vi "Dynamic Dispatch Tester.vi"() -> ()   [LabVIEW 2010]
uses:
  Aggregate Sound/Aggregate Sound.lvclass
  Sound/Sound.lvclass
  <vilib>/Waveform/WDTOps.llb/WDT Append Waveforms DBL.vi
  Single Tone/Single Tone.lvclass
  Silence/Silence.lvclass
  Recorded Sound/Recorded Sound.lvclass
  Fade/Fade.lvclass
panel:
  out "Appended Waveforms":waveform(dbl)(graph)
  in  "Fade in? (True)":bool=TRUE
  in  "Silence Duration (1 second)":dbl=1.0
  in  "Tone Duration (1 second)":dbl=1.0
  in  "Frequency (500 Hz)":dbl=500.0
  # "Single Tone"
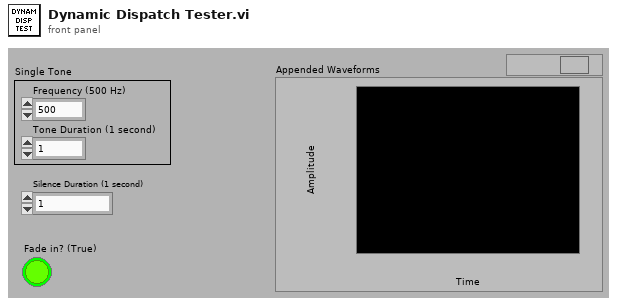
[diagram p1: front panel]
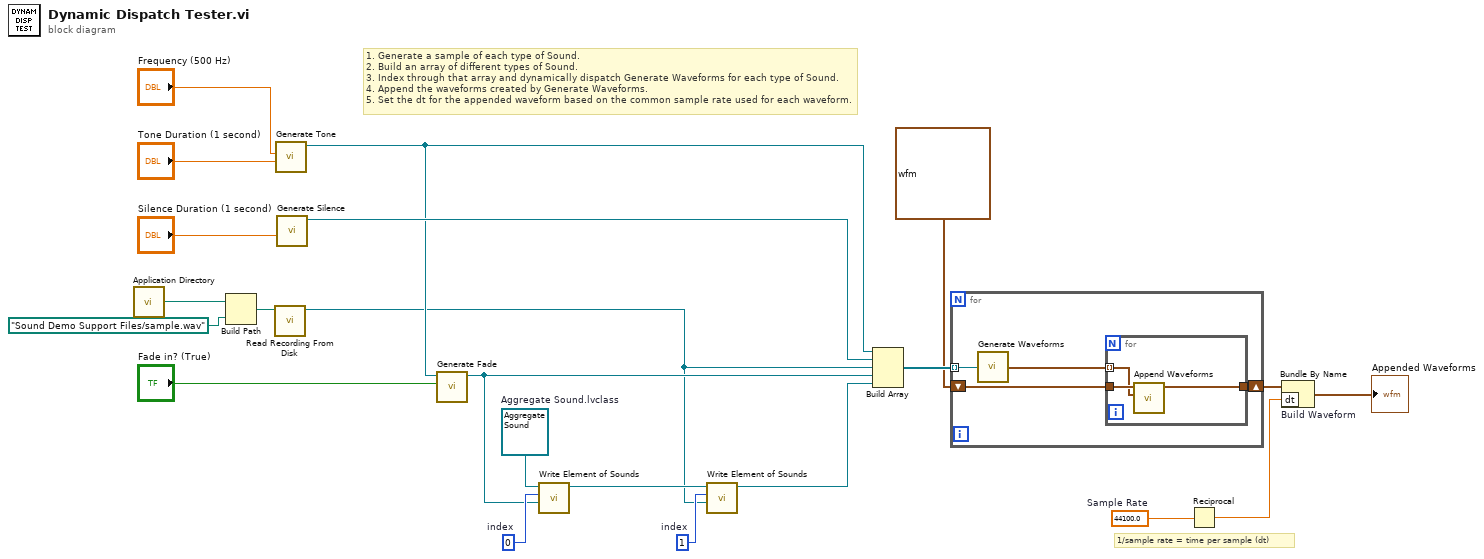
[diagram p0: block diagram]
diagram:
  w10 = 44100.0  # Sample Rate
  w15 = 1  # index
  w16 = 0  # index
  w18 = refnum<class "Aggregate Sound.lvclass"> refnum  # Aggregate Sound.lvclass
  # "1. Generate a sample of each type of Sound. \n2. Build an array of different types of Sound.\n3. Index through that array and dynamically dispatch Generate Waveforms for each type of Sound. \n4. Append the waveforms created by Generate Waveforms.\n5. Set the dt for the appended waveform based on the common sample rate used for each waveform."
  # "1/sample rate = time per sample (dt)"
  n1 = call <vilib>:"Application Directory.vi"() -> ("Application Directory"=w3:path)
  n2 = Build Path(base path=w3, name or relative path=path "Sound Demo Support Files/sample.wav" ("Recorded Sound Path")) -> (appended path=w1:path)
  n3 = call "Read Recording From Disk.vi"("File Path"=w1) -> ("Recorded Sound"=w4:refnum<class "Recorded Sound.lvclass">)  [unwired: 9 in, 1 out]
  n4 = call "Generate Tone.vi"("Duration (1 second)"="Tone Duration (1 second)", "Frequency (500 Hz)"="Frequency (500 Hz)") -> ("Single Tone out"=w5:refnum<class "Single Tone.lvclass">)  [unwired: 9 in]
  n5 = call "Generate Silence.vi"("Duration (1 second)"="Silence Duration (1 second)") -> ("Silence out"=w13:refnum<class "Silence.lvclass">)  [unwired: 10 in]
  n6 = call "Generate Fade.vi"("Fade in? (True)"="Fade in? (True)", "Original Sound"=w5) -> ("Fade"=w7:refnum<class "Fade.lvclass">)  [unwired: 9 in]
  n7 = call "Write Element of Sounds.vi"("Sound.lvclass"=w7, "index"=w16, "Aggregate Sound in"=w18) -> ("Aggregate Sound out"=w17:refnum<class "Aggregate Sound.lvclass">)  [unwired: 8 in]
  n8 = call "Write Element of Sounds.vi"("Sound.lvclass"=w4, "index"=w15, "Aggregate Sound in"=w17) -> ("Aggregate Sound out"=w6:refnum<class "Aggregate Sound.lvclass">)  [unwired: 8 in]
  n9 = Build Array "Build Array"(w5, w13, w4, w7, w6) -> (w14:refnum<class "Sound.lvclass">[])
  n10 = for {
    tunnel: w14 -> [w26] mode=indexing
    shift-right: [w24] -> w11
    shift-left: waveform(dbl) {"t0"=timestamp(0 s since 1904-01-01), "dt"=1.0, "Y"=[]} ("waveform out") -> [w23]
    n11 = call-dynamic "Generate Waveforms.vi"("Sound.lvclass"=w26) -> ("Waveforms"=w25:waveform(dbl)[])
    n12 = for {
      tunnel: w25 -> [w27] mode=indexing
      tunnel: [w29] -> w24
      tunnel: w23 -> [w28]
      n13 = call-poly <vilib>:"Append Waveforms.vi"("waveform B"=w27, "waveform A"=w28) -> ("waveform out"=w29:waveform(dbl))  [unwired: 8 in, 1 out]
    }
  }
  n14 = Reciprocal(x=w10) -> (1/x=w9:dbl)
  n15 = Bundle By Name "Build Waveform"(cluster=w11, "dt"=w9) -> (→"Appended Waveforms":waveform(dbl))
